vi "Zarlink Telemetry.vi"(8 "error in (no error)":errorcluster, 10 "Input":T3={"Command"=enum."Get xPG Status", "Function"=enum."Downlink Only", "MICS_ID"=0, "EXID"=16773121, "Use Local"=FALSE, "Transceive Delay mS"=200.0, "CP_DATA IN"=[], "Parameters"=""} {"Transceive Delay mS" min=0.0 max=10000.0 step=1.0; "EXID" step=1 format="%.0x"; "MICS_ID" step=1 format="%06x"}, 11 "MICS Dongle Address":refnum<visa-resource-name>="COM5") -> (0 "error out":errorcluster, 1 "Status Flags":T1, 2 "Output":T4)   [LabVIEW 2020]
uses:
  Typedef Command List.ctl
  <vilib>/Instr/_visa.llb/VISA Configure Serial Port (Instr).vi
  MICS_ID Global.vi
  MICS_Channel Global.vi
  <vilib>/Utility/file.llb/Write To Spreadsheet File (string).vi
panel:
  in  "MICS Channel (Local)":u16=2
  in  "Use MICS Dongle":bool=TRUE
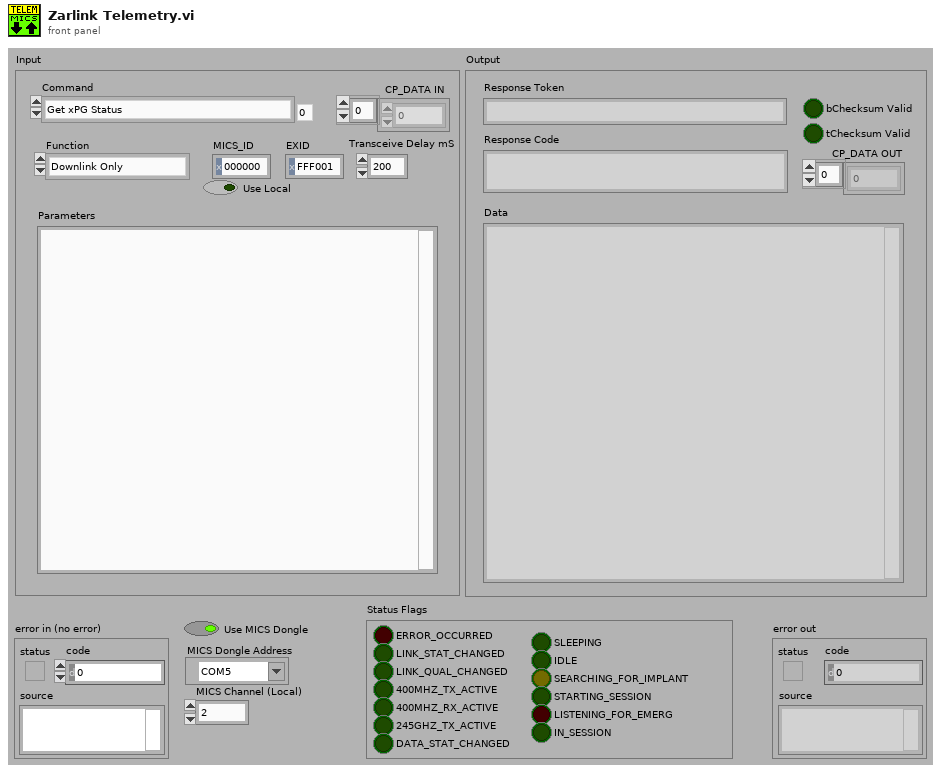
[diagram p1: front panel]
types:
  T1 = cluster{"ERROR_OCCURRED":bool, "LINK_STAT_CHANGED":bool, "LINK_QUAL_CHANGED":bool, "400MHZ_TX_ACTIVE":bool, "400MHZ_RX_ACTIVE":bool, "245GHZ_TX_ACTIVE":bool, "DATA_STAT_CHANGED":bool, "SLEEPING":bool, "IDLE":bool, "SEARCHING_FOR_IMPLANT":bool, "STARTING_SESSION":bool, "LISTENING_FOR_EMERG":bool, "IN_SESSION":bool}
  T2 = typedef "Typedef Command List.ctl" = enum16{"Get xPG Status", "xPG Stimulation", "Select Program", "Increment Program Amplitude", "Decrement Program Amplitude", "Get PoP Constants", "Get PPC Constants", "Get Program Names", "Set Pulse Amplitude", "Increment Pulse Amplitude", "Decrement Pulse Amplitude", "Get Pulse Widths", "Set Pulse Widths", "Increment Pulse Width", "Decrement Pulse Width", "Get Program Frequency", "Set Program Frequency", "Increment Program Frequency", "Decrement Program Frequency", "Inject Event", "Charging Control", "Get xPG Identity", "Set xPG Identity", "Restore Program Defaults", "Get Program Definition", "Set Program Definition", "Get Program Constants", "Set Program Constants", "Get Configurable Device Parameters", "Set Configurable Device Parameters", "Get Pulse Constants", "Set Pulse Constants", "Get Lead Limits", "Set Lead Limits", "Get Channel Calibrations", "Set Channel Calibrations", "<reserved 2>", "<reserved 3>", "<reserved 4>", "<reserved 5>", "<reserved 6>", "<reserved 7>", "Get Stim Asic HV Calibrations", "Set Stim Asic HV Calibrations", "<reserved 8>", "<reserved 9>", "Get CP Data", "Set CP Data", "Clear Log", "Read Log", "Append Log", "Get Patient Program Runtime", "Set Patient Program Runtime", "Impedance Measurement", "Enter Storage Mode", "Echo Short", "Echo Long", "Get General Calibration", "Set General Calibration", "Get Trim List", "Set Trim List", "Get Counter", "Set Counter", "Get Test Stimulation", "Set Test Stimulation", "Get Titration Stimulation", "Set Titration Stimulation", "Get Ramp Time", "Set Ramp Time", "Get VBAT", "Set Software Description Block", "Get Software Description Block", "Write Memory", "Read Memory", "Reset xPG", "Erase Flash Block", "Write Vectors", "Read Vectors", "Diagnostic Data", "Set Background Impedance", "Get Background Impedence ", "Set Test Waveform", "Calibrate Channel", "Get Log Range", "Reserved 0x55", "Reserved 0x56", "MICS Options", "Pair PPC", "Pair POP", "Stop Bootloader", "Tune MICS", "MICS Diagnostics", "Undefined"}
  T3 = cluster{"Command":T2, "Function":enum16{"Open Session", "Close Session", "Downlink Only", "Uplink Only", "Transceive (DN -> UP)"}, "MICS_ID":u32, "EXID":u32, "Use Local":bool, "Transceive Delay mS":dbl, "CP_DATA IN":u8[], "Parameters":string}
  T4 = cluster{"Response Token":string, "Response Code":string, "bChecksum Valid":bool, "tChecksum Valid":bool, "CP_DATA OUT":u8[], "Data":string}
  T5 = cluster{"ConfigFlags":u8, "ImplantID":u32, "CompanyID":u8, "Normal_Comm":cluster{"RF_Channel":u8, "UserData":u8, "TX_Mod":u8, "RX_Mod":u8, "RX_BlockSize":u8, "BlockPerPack":u8, "TX_BlockSize":u8}, "Emerg_Comm":cluster{"RF_Channel":u8, "UserData":u8, "TX_Mod":u8, "RX_Mod":u8, "TX_BlockSize":u8, "BlockPerPack":u8, "RX_BlockSize":u8}, "ImplantRev":u8, "245TX_PowerCal":i8, "245TX_Power":i8, "CCA_RSSI_Thresholds":cluster{"ch0":u16, "ch1":u16, "ch2":u16, "ch3":u16, "ch4":u16, "ch5":u16, "ch6":u16, "ch7":u16, "ch8":u16, "ch9":u16}}
  T6 = enum16{"Open Session", "Close Session", "Downlink Only", "Uplink Only", "Transceive (DN -> UP)"}
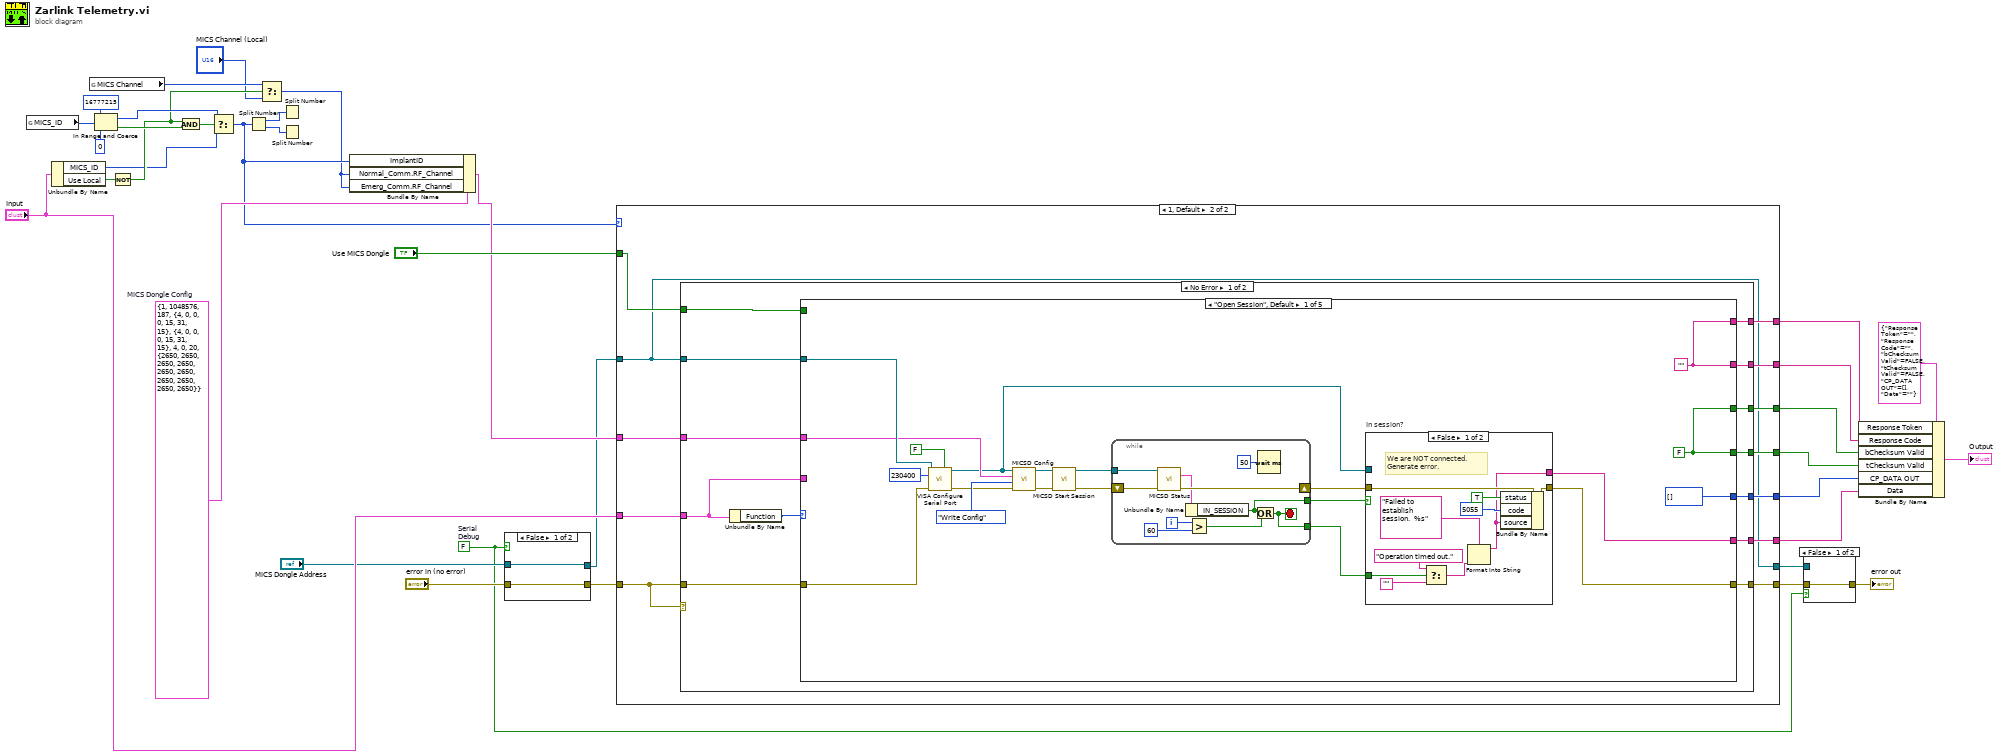
[diagram p0: block diagram]
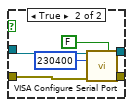
[diagram p2: hidden frame]
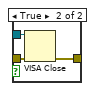
[diagram p3: hidden frame]
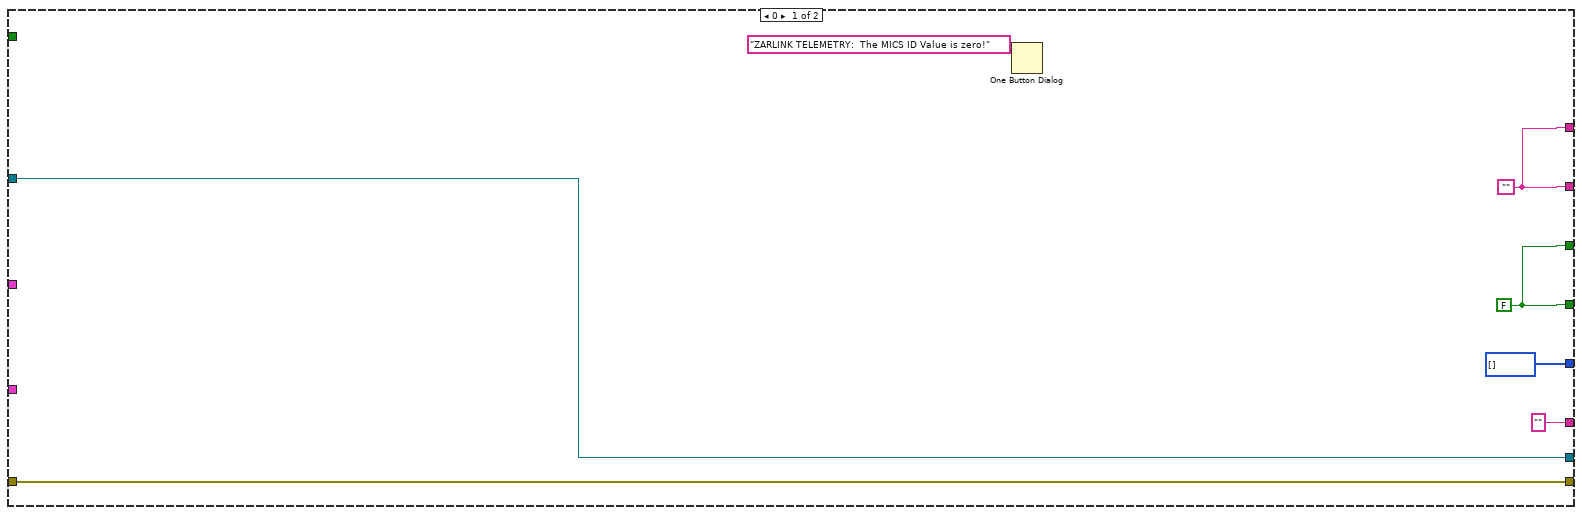
[diagram p4: hidden frame]
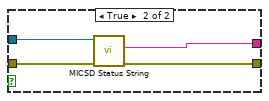
[diagram p5: hidden frame]
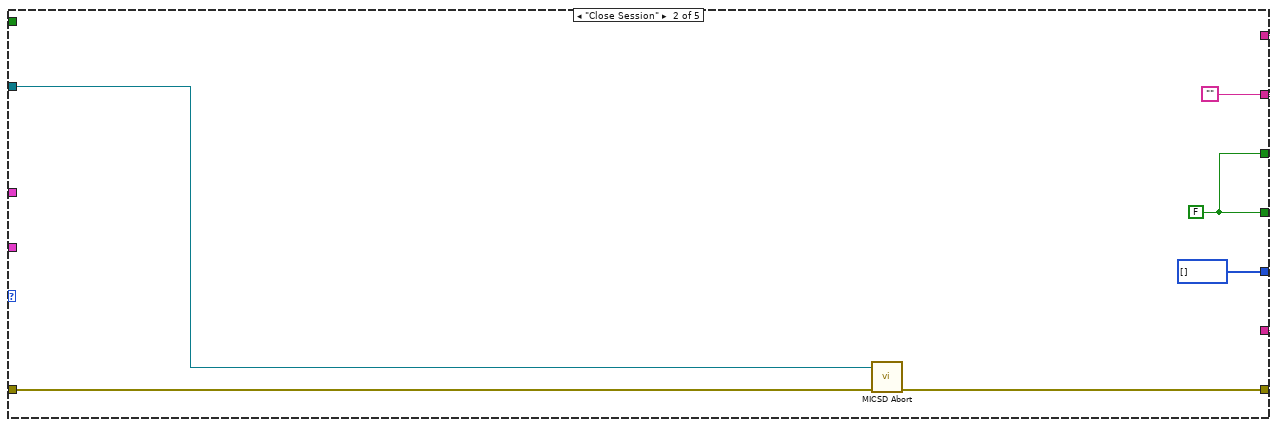
[diagram p6: hidden frame]
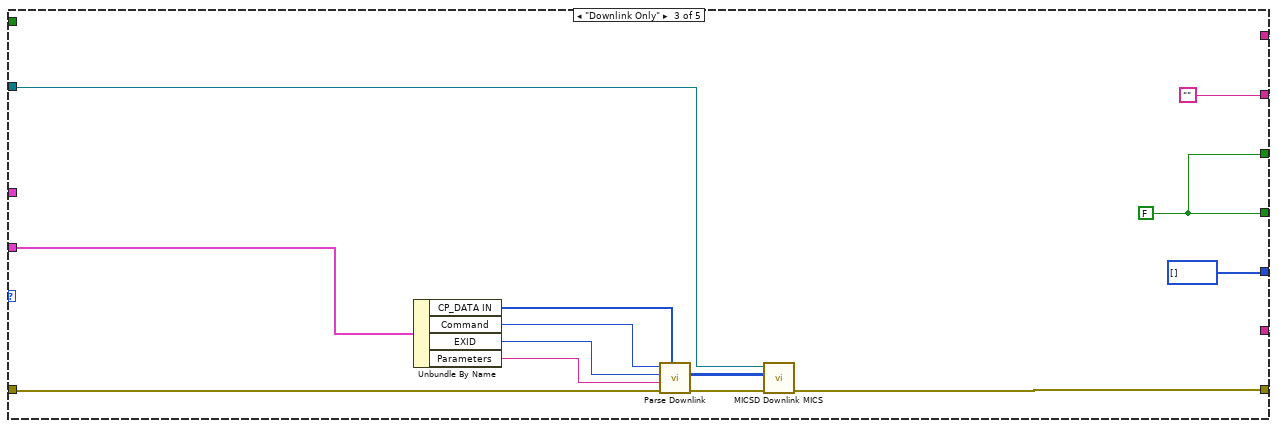
[diagram p7: hidden frame]
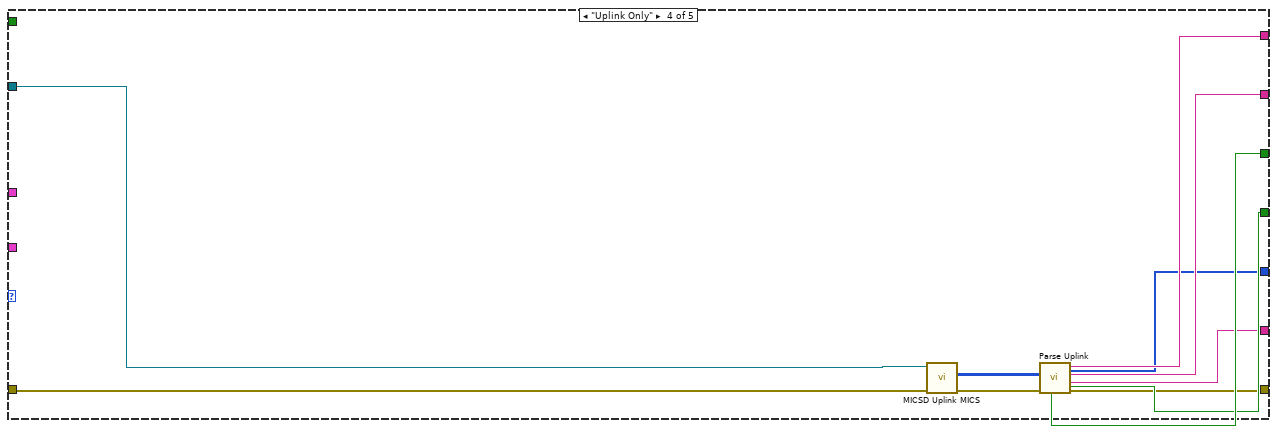
[diagram p8: hidden frame]
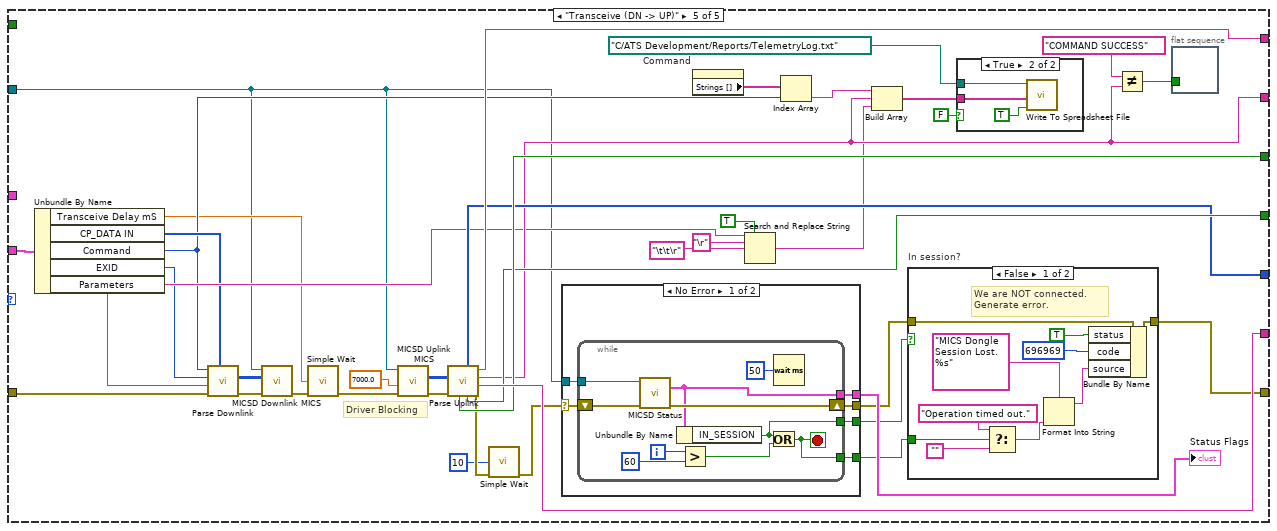
[diagram p9: hidden frame]
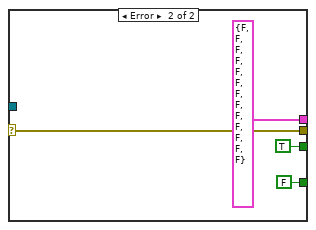
[diagram p10: hidden frame]
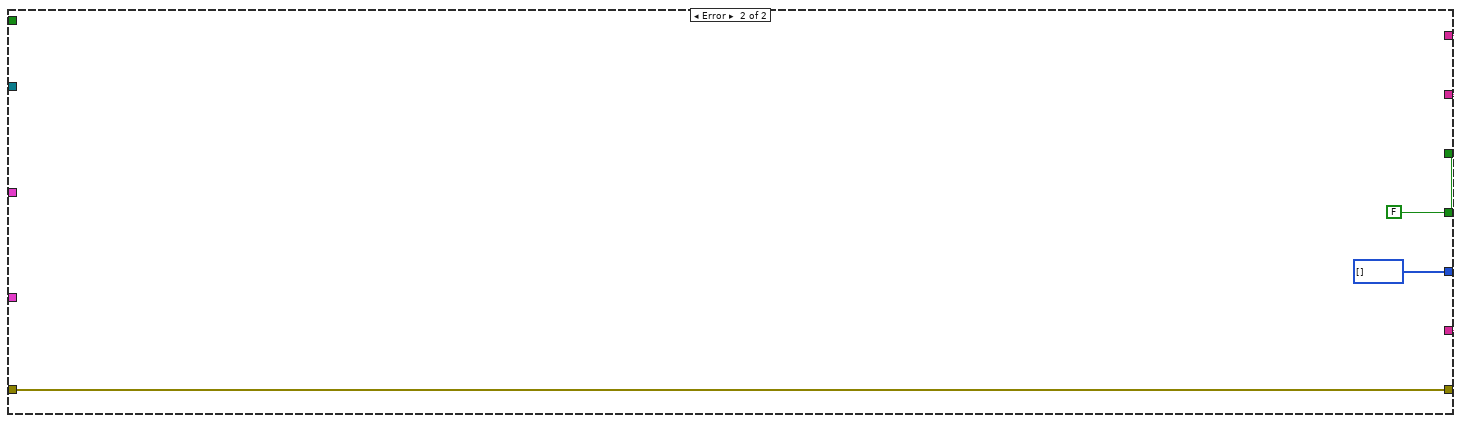
[diagram p13: hidden frame]
diagram:
  w2 = FALSE  # Serial  Debug
  w24 = T5 {"ConfigFlags"=1, "ImplantID"=1048576, "CompanyID"=187, "Normal_Comm"={"RF_Channel"=4, "UserData"=0, "TX_Mod"=0, "RX_Mod"=0, "RX_BlockSize"=15, "BlockPerPack"=31, "TX_BlockSize"=15}, "Emerg_Comm"={"RF_Channel"=4, "UserData"=0, "TX_Mod"=0, "RX_Mod"=0, "TX_BlockSize"=15, "BlockPerPack"=31, "RX_BlockSize"=15}, "ImplantRev"=4, "245TX_PowerCal"=0, "245TX_Power"=20, "CCA_RSSI_Thresholds"={"ch0"=2650, "ch1"=2650, "ch2"=2650, "ch3"=2650, "ch4"=2650, "ch5"=2650, "ch6"=2650, "ch7"=2650, "ch8"=2650, "ch9"=2650}}  # MICS Dongle Config
  n1 = global read "MICS_ID Global.vi" "MICS_ID"() -> (w33:u32)
  n2 = Unbundle By Name("Input") -> ("MICS_ID"=w11:u32, "Use Local"=w12:bool)
  n3 = global read "MICS_Channel Global.vi" "MICS Channel"() -> (w27:u16)
  n4 = In Range and Coerce(upper limit=u32 16777215, x=w33, lower limit=u32 0) -> (coerced(x)=w28:u32, In Range?=w30:bool)
  n5 = Not(x=w12) -> (.not. x?=w26:bool)
  n6 = And(x=w26, y=w30) -> (x .and. y?=w29:bool)
  n7 = Select(t=w28, s=w29, f=w11) -> (s? t:f=w22:u32)
  n8 = Split Number(x=w22) -> (hi(x)=w35:u16, lo(x)=w34:u16)
  n9 = Select(t=w27, s=w26, f="MICS Channel (Local)") -> (s? t:f=w21:u16)
  n10 = Split Number(x=w35) -> ()  [unwired: 2 out]
  n11 = Split Number(x=w34) -> ()  [unwired: 2 out]
  n12 = Bundle By Name(cluster=w24, "ImplantID"=w22, "Normal_Comm.RF_Channel"=w21, "Emerg_Comm.RF_Channel"=w21) -> (w23:T5)
  n13 = case shown="False" w2 {
    tunnel: [w37 w41] -> w9
    tunnel: "error in (no error)" -> [w37 w40]
    tunnel: "MICS Dongle Address" -> [w36 w39]
    tunnel: [w36 w38] -> w6
    frame False {
    }
    frame True {
      n14 = call-poly "VISA Configure Serial Port"("VISA resource name"=w39, "Enable Termination\nChar (T)"=FALSE ("Enable Termination\nChar (T)"), "baud rate (9600)"=u32 230400, "error in (no error)"=w40) -> ("VISA resource name out"=w38:refnum<visa-resource-name>, "error out"=w41:errorcluster)  [unwired: 10 in]
    }
  }
  n15 = case shown="1, Default" w22 {
    tunnel: [w45 w62] -> w5
    tunnel: w9 -> [w45 w61]
    tunnel: [w47 w60] -> w18
    tunnel: [w47 w59] -> w17
    tunnel: [w48 w58] -> w15
    tunnel: [w48 w57] -> w14
    tunnel: [u8[] [] ("CP_DATA OUT") w56] -> w13
    tunnel: ["" ("Data") w55] -> w16
    tunnel: w6 -> [w44 w51]
    tunnel: "Use MICS Dongle" -> [_ w54]
    tunnel: w23 -> [_ w53]
    tunnel: "Input" -> [_ w52]
    tunnel: [w44 w51] -> w3
    frame 0 {
      w47 = ""
      w48 = FALSE
      n16 = One Button Dialog(message="ZARLINK TELEMETRY:  The MICS ID Value is zero!") -> ()  [unwired: 1 in, 1 out]
    }
    frame 1, Default {
      n17 = case shown="No Error" w61 {
        tunnel: w61 -> [w75 w227]
        tunnel: [w74 w227] -> w62
        tunnel: [w68 w224] -> w60
        tunnel: [w69 w224] -> w59
        tunnel: [w70 w226] -> w58
        tunnel: [w71 w226] -> w57
        tunnel: [w72 u8[] [] ("CP_DATA OUT")] -> w56
        tunnel: [w73 w224] -> w55
        tunnel: w51 -> [w67 _]
        tunnel: w54 -> [w66 _]
        tunnel: w53 -> [w65 _]
        tunnel: w52 -> [w63 _]
        frame No Error {
          n18 = Unbundle By Name(w63) -> ("Function"=w64:T6)
          n19 = case shown="\"Open Session\", Default" w64 {
            tunnel: w75 -> [w90 w123 w136 w140 w188]
            tunnel: [w91 w122 w132 w141 w154] -> w74
            tunnel: [w92 w121 w133 w142 w186] -> w73
            tunnel: [u8[] [] ("CP_DATA OUT") u8[] [] ("CP_DATA OUT") u8[] [] ("CP_DATA OUT") w143 w182] -> w72
            tunnel: [w95 w124 w135 w144 w183] -> w71
            tunnel: [w95 w124 w135 w145 w184] -> w70
            tunnel: [w94 w121 w133 w146 w174] -> w69
            tunnel: [w94 w121 w133 w147 w185] -> w68
            tunnel: w67 -> [w89 w120 w131 w139 w155]
            tunnel: w66 -> [_ _ _ _ _]
            tunnel: w65 -> [w88 _ _ _ _]
            tunnel: w63 -> [_ _ w130 _ w166]
            frame "Open Session", Default {
              w94 = ""
              w95 = FALSE
              n20 = call-poly "VISA Configure Serial Port"("VISA resource name"=w89, "Enable Termination\nChar (T)"=FALSE ("Enable Termination\nChar (T)"), "baud rate (9600)"=u32 230400, "error in (no error)"=w90) -> ("VISA resource name out"=w77:refnum<visa-resource-name>, "error out"=w78:errorcluster)  [unwired: 10 in]
              n21 = call "MICSD Config.vi"("error in (no error)"=w78, "Function"=enum16{"Write Config", "Read Config"}."Write Config", "MICS_Config_In"=w88, "VISA Resource Name"=w77) -> ("error out"=w86:errorcluster, "dup VISA Resource Name"=w85:refnum<visa-resource-name>)  [unwired: 5 in, 1 out]
              n22 = call "MICSD Start Session.vi"("error in (no error)"=w86, "VISA Resource Name"=w85) -> ("error out"=w76:errorcluster, "dup VISA Resource Name"=w84:refnum<visa-resource-name>)  [unwired: 8 in]
              n23 = while {
                tunnel: w84 -> [w104]
                shift-right: [w103] -> w82
                shift-left: w76 -> [w105]
                tunnel: [w97] -> w83
                tunnel: [w96] -> w81
                i -> [w99]
                stop <- w96 stop-if-true
                n24 = call "MICSD Status.vi"("VISA Resource Name"=w104, "error in (no error)"=w105) -> ("Status Flags"=w102:T1, "error out"=w103:errorcluster)  [unwired: 7 in, 5 out]
                n25 = Unbundle By Name(w102) -> ("IN_SESSION"=w97:bool)
                n26 = Greater?(x=w99, y=60) -> (0:w100:bool)
                n27 = Or(x=w97, y=w100) -> (x .or. y?=w96:bool)
                n28 = Wait (ms)(milliseconds to wait=u32 50) -> ()  [unwired: 1 out]
              }
              n29 = case "In session?" shown="False" w83 {
                tunnel: w82 -> [w115 w119]
                tunnel: [w109 w118] -> w91
                tunnel: w81 -> [w113 _]
                tunnel: [w106 w116] -> w92
                tunnel: w77 -> [_ w117]
                frame False {
                  # "We are NOT connected. Generate error."
                  n30 = Select(t="Operation timed out." ("format string"), s=w113, f="") -> (s? t:f=w108:string)
                  n31 = Format Into String(format string="Failed to establish session.  %s", w108) -> (resulting string=w106:string)  [unwired: 2 in, 1 out]
                  n32 = Bundle By Name(cluster=w115, "status"=TRUE, "code"=5055, "source"=w106) -> (w109:errorcluster)
                }
                frame True {
                  n33 = call "MICSD Status String.vi"("error in (no error)"=w119, "VISA Resource Name"=w117) -> ("error out"=w118:errorcluster, "Response"=w116:string)  [unwired: 7 in, 1 out]
                }
              }
            }
            frame "Close Session" {
              w121 = ""
              w124 = FALSE
              n34 = call "MICSD Abort.vi"("error in (no error)"=w123, "VISA Resource Name"=w120) -> ("error out"=w122:errorcluster)  [unwired: 8 in, 1 out]
            }
            frame "Downlink Only" {
              w133 = ""
              w135 = FALSE
              n35 = Unbundle By Name(w130) -> ("CP_DATA IN"=w129:u8[], "Command"=w128:T2, "EXID"=w127:u32, "Parameters"=w126:string)
              n36 = call "Parse Downlink.vi"("CP_DATA IN"=w129, "error in (no error)"=w136, "Parameters"=w126, "EXID"=w127, "Command"=w128) -> ("error out"=w138:errorcluster, "Downlink"=w137:u8[][])  [unwired: 5 in]
              n37 = call "MICSD Downlink MICS.vi"("Error In"=w138, "Downlink"=w137, "VISA Resource Name"=w131) -> ("Error Out"=w132:errorcluster)  [unwired: 7 in, 1 out]
            }
            frame "Uplink Only" {
              n38 = call "MICSD Uplink MICS.vi"("Error In"=w140, "VISA Resource Name"=w139) -> ("Error Out"=w149:errorcluster, "Uplink"=w148:u8[][])  [unwired: 7 in, 1 out]
              n39 = call "Parse Uplink.vi"("error in (no error)"=w149, "Uplink"=w148) -> ("error out"=w141:errorcluster, "Data"=w142:string, "Response Code"=w146:string, "Response Token"=w147:string, "tChecksum Valid"=w144:bool, "CP_DATA"=w143:u8[], "bChecksum Valid"=w145:bool)  [unwired: 3 in]
            }
            frame "Transceive (DN -> UP)" {
              # "Driver Blocking"
              n40 = Unbundle By Name(w166) -> ("Transceive Delay mS"=w158:dbl, "CP_DATA IN"=w164:u8[], "Command"=w162:T2, "EXID"=w163:u32, "Parameters"=w165:string)
              n41 = call "Parse Downlink.vi"("CP_DATA IN"=w164, "error in (no error)"=w188, "Parameters"=w165, "EXID"=w163, "Command"=w162) -> ("error out"=w189:errorcluster, "Downlink"=w161:u8[][])  [unwired: 5 in]
              n42 = call "MICSD Downlink MICS.vi"("Error In"=w189, "Downlink"=w161, "VISA Resource Name"=w155) -> ("Error Out"=w180:errorcluster)  [unwired: 7 in, 1 out]
              n43 = call "Simple Wait.vi"("mS"=w158, "error in"=w180) -> ("error out"=w179:errorcluster)  [unwired: 12 in, 1 out]
              n44 = call "MICSD Uplink MICS.vi"("Error In"=w179, "Timeout(mS)"=7000.0, "VISA Resource Name"=w155) -> ("Error Out"=w187:errorcluster, "Uplink"=w181:u8[][])  [unwired: 6 in, 1 out]
              n45 = call "Parse Uplink.vi"("error in (no error)"=w187, "Uplink"=w181) -> ("error out"=w160:errorcluster, "Data"=w186:string, "Response Code"=w174:string, "Response Token"=w185:string, "tChecksum Valid"=w183:bool, "CP_DATA"=w182:u8[], "bChecksum Valid"=w184:bool)  [unwired: 3 in]
              n46 = call "Simple Wait.vi"("mS"=u32 10, "error in"=w160) -> ("error out"=w150:errorcluster)  [unwired: 12 in, 1 out]
              n47 = case shown="No Error" w150 {
                selector: w150 -> [w190 w209]
                tunnel: [w195 T1 {"ERROR_OCCURRED"=FALSE, "LINK_STAT_CHANGED"=FALSE, "LINK_QUAL_CHANGED"=FALSE, "400MHZ_TX_ACTIVE"=FALSE, "400MHZ_RX_ACTIVE"=FALSE, "245GHZ_TX_ACTIVE"=FALSE, "DATA_STAT_CHANGED"=FALSE, "SLEEPING"=FALSE, "IDLE"=FALSE, "SEARCHING_FOR_IMPLANT"=FALSE, "STARTING_SESSION"=FALSE, "LISTENING_FOR_EMERG"=FALSE, "IN_SESSION"=FALSE} ("Status Flags")] -> w156
                tunnel: w155 -> [w194 _]
                tunnel: [w193 TRUE ("IN_SESSION")] -> w153
                tunnel: [w192 FALSE] -> w152
                tunnel: [w191 w209] -> w151
                frame No Error {
                  n48 = while {
                    tunnel: w194 -> [w204]
                    shift-right: [w203] -> w191
                    shift-left: w190 -> [w205]
                    tunnel: [w198] -> w193
                    tunnel: [w197] -> w192
                    tunnel: [w196] -> w195
                    i -> [w200]
                    stop <- w197 stop-if-true
                    n49 = call "MICSD Status.vi"("VISA Resource Name"=w204, "error in (no error)"=w205) -> ("Status Flags"=w196:T1, "error out"=w203:errorcluster)  [unwired: 7 in, 5 out]
                    n50 = Unbundle By Name(w196) -> ("IN_SESSION"=w198:bool)
                    n51 = Greater?(x=w200, y=60) -> (0:w201:bool)
                    n52 = Or(x=w198, y=w201) -> (x .or. y?=w197:bool)
                    n53 = Wait (ms)(milliseconds to wait=u32 50) -> ()  [unwired: 1 out]
                  }
                }
                frame Error {
                }
              }
              "Status Flags" <- w156
              n54 = property on="Command" class="Enum (strict)"() -> ("Strings []"=w176:string[])  [unwired: 2 in, 2 out]
              n55 = Search and Replace String(replace all?=TRUE ("replace all? (F)"), input string=w165, search string="\r", replace string="\t\t\r" ("search string")) -> (result string=w171:string)  [unwired: 4 in, 3 out]
              n56 = Index Array(array=w176, index=w162) -> (element=w175:string)
              n57 = Build Array(w175, w174, w171) -> (w172:string[])
              n58 = case "In session?" shown="False" w153 {
                tunnel: w151 -> [w210 w220]
                tunnel: [w214 w220] -> w154
                tunnel: w152 -> [w218 _]
                frame False {
                  # "We are NOT connected. Generate error."
                  n59 = Select(t="Operation timed out." ("format string"), s=w218, f="") -> (s? t:f=w213:string)
                  n60 = Format Into String(format string="MICS Dongle Session Lost.  %s", w213) -> (resulting string=w211:string)  [unwired: 2 in, 1 out]
                  n61 = Bundle By Name(cluster=w210, "status"=TRUE, "code"=696969, "source"=w211) -> (w214:errorcluster)
                }
                frame True {
                }
              }
              n62 = case shown="True" FALSE {
                tunnel: path "C:/ATS Development/Reports/TelemetryLog.txt" ("file (use dialog)") -> [_ w223]
                tunnel: w172 -> [_ w222]
                frame False {
                }
                frame True {
                  n63 = call-poly <vilib>:"Write To Spreadsheet File.vi"("append to file? (new file:F)"=TRUE, "1D data"=w222, "file path (dialog if empty)"=w223) -> ()  [unwired: 5 in, 1 out]
                }
              }
              n64 = Not Equal?(x="COMMAND SUCCESS", y=w174) -> (x != y?=w177:bool)
              n65 = flat-sequence {
                tunnel: w177 -> [_]
                frame #0 {
                }
              }
            }
          }
        }
        frame Error {
          w224 = ""
          w226 = FALSE
        }
      }
    }
  }
  n66 = case shown="False" w2 {
    tunnel: w5 -> [w228 w231]
    tunnel: [w228 w230] -> w4
    tunnel: w3 -> [_ w229]
    frame False {
    }
    frame True {
      n67 = VISA Close(VISA resource name=w229, error in (no error)=w231) -> (error out=w230:errorcluster)
    }
  }
  "error out" <- w4
  n68 = Bundle By Name(cluster=T4 {"Response Token"="", "Response Code"="", "bChecksum Valid"=FALSE, "tChecksum Valid"=FALSE, "CP_DATA OUT"=[], "Data"=""} ("Output"), "Response Token"=w18, "Response Code"=w17, "bChecksum Valid"=w15, "tChecksum Valid"=w14, "CP_DATA OUT"=w13, "Data"=w16) -> (→"Output":T4)
